vi "Write hours.vi"(8 "error in (no error)":errorcluster, 10 "hours":dbl[unit] min=0.0 max=86400.0, 11 "ClockTimes in":refnum<class "ClockTimes.lvclass">) -> (0 "error out":errorcluster, 3 "ClockTimes out":refnum<class "ClockTimes.lvclass">)   [LabVIEW 2014, in "TCSDataDefinitions.lvlib" / "TCSPublicStatus.lvlib" / "CurrentTimes.lvlib" / "ClockTimes.lvclass"]
uses:
  ClockTimes.lvclass
  ClockTimes.lvclass/ClockTimes.ctl
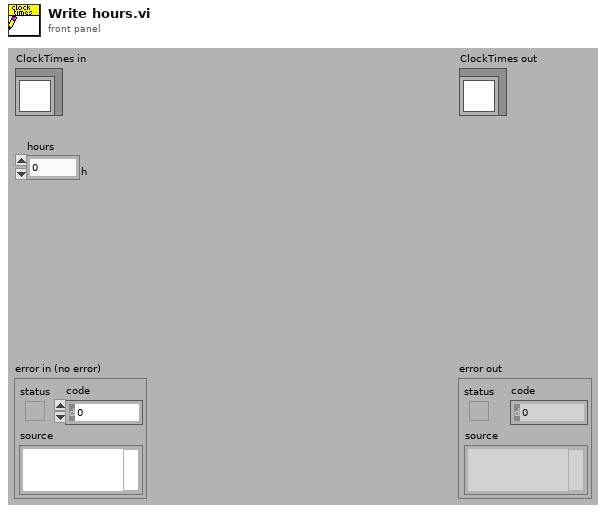
[diagram p1: front panel]
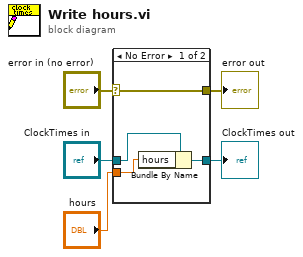
[diagram p0: block diagram]
diagram:
  n1 = case shown="No Error" "error in (no error)" {
    selector: "error in (no error)" -> [w9 w10]
    tunnel: [w9 w10] -> w4
    tunnel: [w7 w11] -> w2
    tunnel: "ClockTimes in" -> [w8 w11]
    tunnel: "hours" -> [w6 _]
    frame No Error {
      n2 = Bundle By Name(cluster=w8, "hours"=w6) -> (w7:refnum<class "ClockTimes.lvclass">)
    }
    frame Error {
    }
  }
  "error out" <- w4
  "ClockTimes out" <- w2
